vi "Set Magnet Field.vi"(4 "Mode":T2, 6 "Axis":T1, 8 "error in (no error)":errorcluster, 9 "Target Rate (T/min)":dbl, 10 "Target Field (T)":dbl, 11 "instrument.PPMS in":refnum<class "instrument.PPMS3.lvclass">) -> (0 "error out":errorcluster, 3 "instrument.PPMS out":refnum<class "instrument.PPMS3.lvclass">)   [LabVIEW 2016, in "instrument.PPMS3.lvclass"]
uses:
  instrument.PPMS3.lvclass
  <userlib>/LevyLab/Levylab Instruments/Instrument Types/Cryostat/Typedefs/Magnet Mode--Enum.ctl
  <userlib>/LevyLab/Levylab Instruments/Instrument Types/Cryostat/Typedefs/Magnet Axis--Enum.ctl
  Typedefs/PPMS3.Commands-enum.ctl
  instrument.PPMS/Typedefs/PPMS.Magnet Field--cluster.ctl
  <userlib>/LevyLab/Levylab Instruments/Instrument Types/Cryostat/Instrument.Cryostat.lvclass
  instrument.PPMS/instrument.PPMS.lvclass
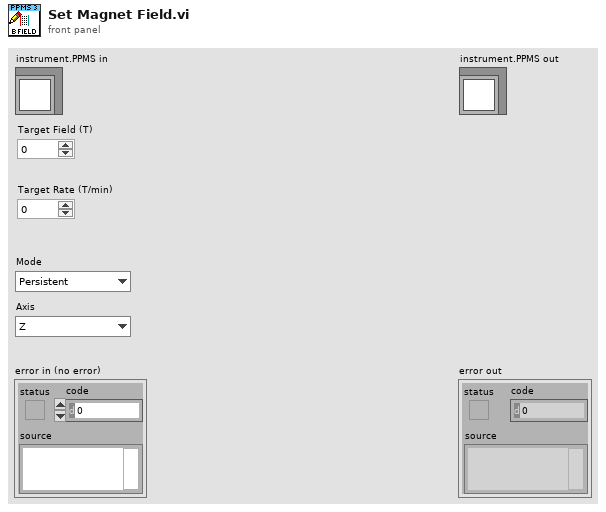
[diagram p1: front panel]
types:
  T1 = typedef "Instrument.Cryostat.lvclass/Magnet Axis--Enum.ctl" = enum16{"Z", "X", "Y"}
  T2 = typedef "Instrument.Cryostat.lvclass/Magnet Mode--Enum.ctl" = enum16{"Persistent", "Driven"}
  T3 = typedef "instrument.PPMS.lvclass/PPMS.Magnet Field--cluster.ctl" = cluster{"Target Field (T)":dbl, "Target Rate (T/min)":dbl, "Mode":T2}
  T4 = typedef "instrument.PPMS3.lvclass/PPMS3.Commands-enum.ctl" = enum16{"Get Magnet Field", "Get Helium Level", "Get Temperature", "Set Magnet Field", "Set Temperature", "getAll"}
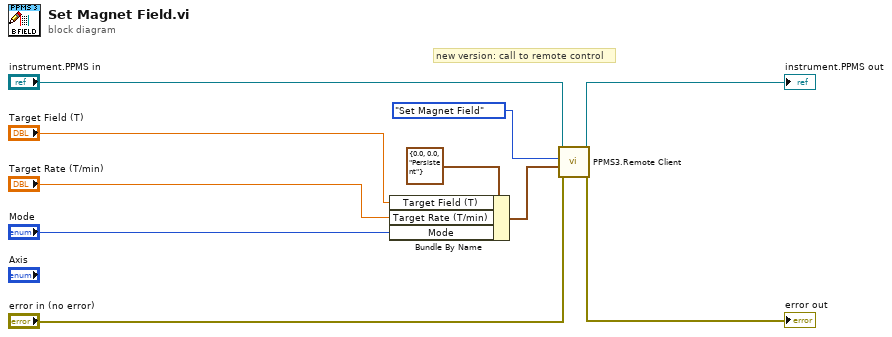
[diagram p0: block diagram]
diagram:
  # "new version: call to remote control"
  n1 = Bundle By Name(cluster=T3 {"Target Field (T)"=0.0, "Target Rate (T/min)"=0.0, "Mode"=enum."Persistent"} ("Magnet Field"), "Target Field (T)"="Target Field (T)", "Target Rate (T/min)"="Target Rate (T/min)", "Mode"="Mode") -> (w3:T3)
  n2 = call "PPMS3.Remote Client.vi"("error in (no error)"="error in (no error)", "Data"=w3, "Command"=PPMS3.Commands-enum."Set Magnet Field", "instrument.PPMS in"="instrument.PPMS in") -> ("error out"=→"error out":errorcluster, "instrument.PPMS out"=→"instrument.PPMS out":refnum<class "instrument.PPMS3.lvclass">)  [unwired: 4 in, 2 out]
